vi "SVFA Zoom Power Spectral Density (N Ch).vi"(0 "scaled signals [EU]":waveform(dbl)[](array[waveform]), 3 "zoom settings":T2={"frequency range"={"start frequency"=1000.0, "stop frequency"=2000.0}, "window"=1, "number of lines"=400, "% overlap"=0.0} {"% overlap" min=0.0 format="%.2f"; "number of lines" min=2; "window" items=["None ", "Hanning", "Hamming", "Blackman-Harris", "Exact Blackman", "Blackman", "Flat Top", "4 Term B-Harris ", "7 Term B-Harris", "Low Sidelobe"]; "frequency range"."stop frequency" min=0.0 format="%.2f"; "frequency range"."start frequency" min=0.0 format="%.2f"}, 4 "dB On (T)":bool=TRUE, 5 "error in (no error)":errorcluster, 6 "desired units":enum16{"EU^2 / Hz", "EU / sqrt(Hz)"}(ring), 7 "averaging parameters":T1={"averaging mode"=enum."No averaging", "weighting mode"=enum."Exponential", "number of averages"=10, "linear mode"=enum."One shot"} {"number of averages" min=1 step=1}, 9 "restart averaging (F)":bool) -> (11 "averaging done":bool, 12 "new spectrum available":bool, 13 "averages completed":dbl, 14 "power spectral densities [EU^2 rms / Hz]":cluster{"f0":dbl, "df":dbl, "magnitude":dbl[]}[](array[cluster]) {"magnitude" format="%.2p"; "df" format="%.2p"; "f0" format="%.2p"}, 15 "unit labels":string[](array[string]), 18 "spectrum info":T3[](array[typedef]) {"x-axis units" items=["Time (s)"=0, "Frequency-CB (Hz)"=1, "Frequency-CPB (Hz)"=1248, "Frequency-Arbitrary (Hz)"=2357, "Quefrency (s)"=2, "Revolutions (rev)"=3, "Order"=4, "Speed (RPM)"=11, "Speed (rad/s)"=21, "Index"=65535]; "weighting filter" items=["Linear", "A-weighting", "B-weighting", "C-weighting", "ITU-R 468-4", "Dolby", "CCITT", "C-message", "Wb", "Wc", "Wd", "We", "Wf", "Wh", "Wj", "Wk", "Wm", "AES17 20 kHz lowpass", "AES17 40 kHz lowpass", "AES17 20 kHz highpass", "AES17 40 kHz highpass"]; "dB reference [EU]" format="%.2f"; "engineering units" items=["custom..."=0, "V"=1, "A"=21, "C"=30, "pC"=31, "s"=32, "-"=29, "Pa"=2, "N"=20, "g"=3, "m/s^2"=4, "m/s"=5, "m"=6, "mm/s"=12, "mm"=13, "micron/s"=14, "micron"=15, "in/s^2"=7, "in/s"=8, "in"=9, "mil/s"=10, "mil"=11, "rad/s^2"=16, "rad/s"=17, "rad"=18, "deg/s^2"=26, "deg/s"=27, "deg"=28, "RPM"=22, "cycle/s^2"=23, "Hz"=24, "cycle"=25, "strain"=19]; "spectral info"."window" items=["None "=0, "Hanning"=1, "Hamming"=2, "Blackman-Harris"=3, "Exact Blackman"=4, "Blackman"=5, "Flat Top"=6, "4 Term B-Harris "=7, "7 Term B-Harris"=8, "Low Sidelobe"=9, "Force - Exponential"=10, "Gaussian"=62]}, 19 "error out":errorcluster)   [LabVIEW 2017]
doc: "Computes the zoom power spectral density of <B>scaled signal [EU]</B> and <B>zoom settings</B>. Data accumulates each time this VI is called. However, it returns a new spectrum only when sufficient data accumulates. Indicators and subsequent processing should only be called when <B>new spectrum available</B> is TRUE. Wire data to the <B>scaled signal [EU]</B> input to determine the polymorphic instance to use or manually select the instance."
uses:
  <vilib>/addons/_NISVFA/_Shared subVIs/Controls/svc_Spectrum Info.ctl
  <vilib>/addons/_NISVFA/_Shared subVIs/Controls/svc_X-Axis Units.ctl
  <vilib>/addons/_NISVFA/_Shared subVIs/Controls/svc_Spectrum Type.ctl
  <vilib>/addons/_NISVFA/_Shared subVIs/Controls/svc_Engineering Units Text Ring.ctl
  <vilib>/addons/_NISVFA/_Shared subVIs/Controls/svc_Weighting Filter Text Ring.ctl
  <vilib>/addons/_NISVFA/_Shared subVIs/Controls/svc_Complimentary Spectrum Units.ctl
  <vilib>/addons/_NISVFA/_Shared subVIs/Spectrum Info/svfa_Build Spectrum Info.vi
  <vilib>/addons/_NISVFA/_Shared subVIs/Spectrum Averaging/svfa_Reset Averaging State Info.vi
  <vilib>/addons/_NISVFA/_Shared subVIs/Spectrum Averaging/svfa_Average Array with Avg Checks (complex) No State.vi
  <vilib>/addons/_NISVFA/_Shared subVIs/Common/svc_Complex to Mag2 Array.vi
  <vilib>/addons/_NISVFA/_Shared subVIs/Spectrum Averaging/svfa_Average Array with Avg Checks (real) No State.vi
  <vilib>/addons/_NISVFA/_Shared subVIs/Common/svc_Get SV Channel Info.vi
  <vilib>/addons/_NISVFA/_Shared subVIs/Common/svc_Spectrum Units.vi
  <vilib>/addons/_NISVFA/_Shared subVIs/Spectrum Averaging/svfa_Average Array (complex) No State.vi
  <vilib>/addons/_NISVFA/_Shared subVIs/Spectrum Averaging/svfa_Average Array (real) No State.vi
  <vilib>/addons/_NISVFA/_Shared subVIs/Spectrum Averaging/svfa_No Average Array (complex).vi
  <vilib>/addons/_NISVFA/_Shared subVIs/Spectrum Averaging/svfa_Average Array (complex).vi
  <vilib>/addons/_NISVFA/_Shared subVIs/Spectrum Averaging/svfa_No Average Array (real).vi
  <vilib>/addons/_NISVFA/_Shared subVIs/Spectrum Averaging/svfa_Average Array (real).vi
  <vilib>/addons/_NISVFA/_Shared subVIs/Spectrum Averaging/svfa_Peak Hold Array.vi
  <vilib>/addons/_NISVFA/_Spectrum Processing/SVFA Unit Conversion (N Ch).vi
  <vilib>/addons/_NISVFA/_Shared subVIs/Common/svc_Get Weighting Enum and Labels.vi
  <vilib>/addons/_NISVFA/_Shared subVIs/Common/svc_Unit Label Lexical Class.vi
  <vilib>/addons/_NISVFA/_Shared subVIs/Common/svc_Engineering Units to Unit Label.vi
  <vilib>/addons/_NISVFA/_Shared subVIs/Common/svc_Format Value (DBL).vi
  <vilib>/addons/_NISVFA/_Shared subVIs/Common/svc_Channel Info to Spectrum Info.vi
  <vilib>/addons/_NISVFA/_Shared subVIs/Common/svc_Unit Label to Engineering Units.vi
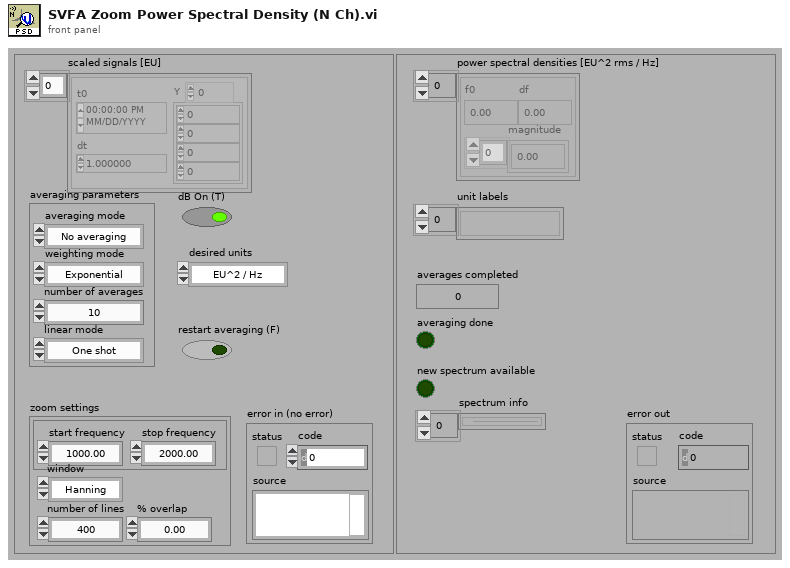
[diagram p1: front panel]
types:
  T1 = cluster{"averaging mode":enum16{"No averaging", "Vector averaging", "RMS averaging", "Peak hold"}, "weighting mode":enum16{"Linear", "Exponential"}, "number of averages":u32, "linear mode":enum16{"One shot", "Auto restart"}}
  T2 = cluster{"frequency range":cluster{"start frequency":dbl, "stop frequency":dbl}, "window":u16, "number of lines":i32, "% overlap":dbl}
  T3 = typedef "svc_Spectrum Info.ctl" = cluster{"channel name":string, "description":string, "x-axis units":T4, "spectral info":cluster{"spectrum type":T5, "linear/dB":enum16{"linear", "dB"}, "window":u16, "window size":i32, "FFT size":i32}, "engineering units":T6, "custom label":string, "dB reference [EU]":dbl, "peak units":enum16{"rms", "peak", "peak-peak"}, "weighting filter":T7, "spectral density?":bool, "unit label":string, "spectrum skewed?":bool, "complimentary spectrum units":T8}
  T4 = typedef "svc_X-Axis Units.ctl" = u16
  T5 = typedef "svc_Spectrum Type.ctl" = enum16{"FFT Spectrum [complex]", "Amplitude [Magnitude]", "Power [Magnitude^2]", "Cross Spectrum [complex]", "Frequency Response [Complex]"}
  T6 = typedef "svc_Engineering Units Text Ring.ctl" = u16
  T7 = typedef "svc_Weighting Filter Text Ring.ctl" = u16
  T8 = typedef "svc_Complimentary Spectrum Units.ctl" = enum16{"none", "radians", "degrees", "cycles", "imaginary"}
  T9 = enum16{"Restart processing", "Continue processing", "Skip processing"}
  T10 = enum16{"No averaging", "Vector averaging", "RMS averaging", "Peak hold"}
  T11 = cluster{"linear/dB":enum16{"no change", "linear", "dB"}, "dB reference (0: no change)":dbl, "power/magnitude":enum16{"no change", "power", "magnitude"}, "view":enum16{"no change", "rms", "peak", "peak-peak"}}
  T12 = enum16{"no change", "spectrum", "spectral density"}
  T13 = cluster{"zoom settings":cluster{"center frequency":dbl, "zoom":i32, "trim":dbl}, "FFT settings":cluster{"window":enum16{"None ", "Hanning", "Hamming", "Blackman-Harris", "Exact Blackman", "Blackman", "Flat Top", "4 Term B-Harris ", "7 Term B-Harris", "Low Sidelobe"}, "window size":i32, "FFT size":i32, "%overlap":dbl}}
  T14 = cluster{"complex FFT":cdb[], "real FFT":dbl[], "f0":dbl, "df":dbl, "averages completed":dbl, "averaging parameters":cluster{"averaging mode":enum16{"No averaging", "Vector averaging", "RMS averaging", "Peak hold"}, "weighting mode":enum16{"Linear", "Exponential"}, "number of averages":u32, "linear mode":enum16{"One shot", "Auto restart"}}}[]
  T15 = cluster{"complex FFT":cdb[], "real FFT":dbl[], "f0":dbl, "df":dbl, "averages completed":dbl, "averaging parameters":cluster{"averaging mode":enum16{"No averaging", "Vector averaging", "RMS averaging", "Peak hold"}, "weighting mode":enum16{"Linear", "Exponential"}, "number of averages":u32, "linear mode":enum16{"One shot", "Auto restart"}}}
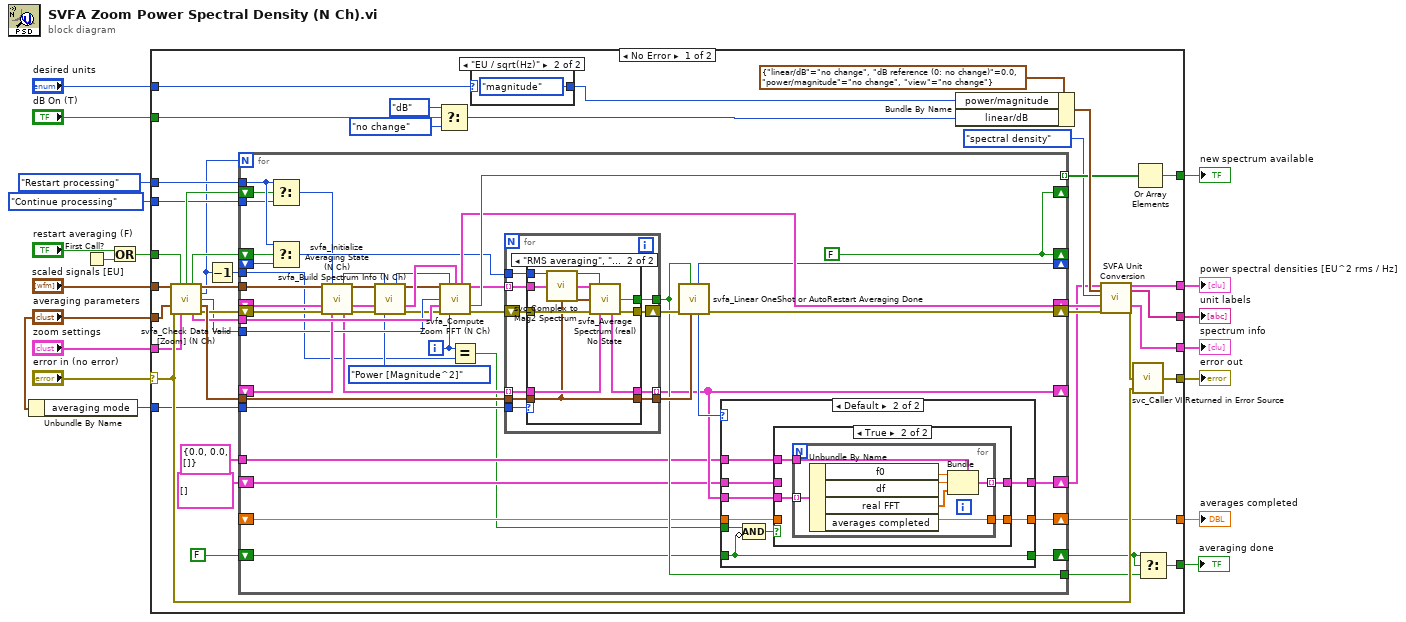
[diagram p0: block diagram]
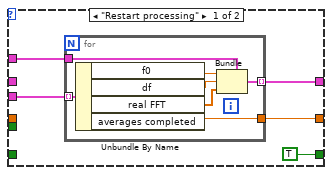
[diagram p2: hidden frame]
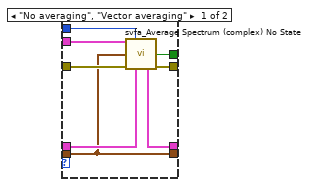
[diagram p4: hidden frame]
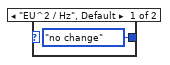
[diagram p5: hidden frame]
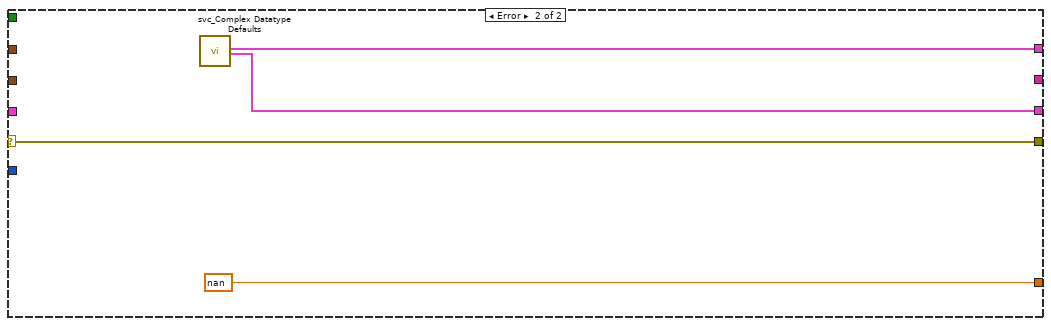
[diagram p6: hidden frame]
diagram:
  n1 = Unbundle By Name("averaging parameters") -> ("averaging mode"=w1:T10)
  n2 = First Call?() -> (First Call?: T/F=w8:bool)
  n3 = Or(x="restart averaging (F)", y=w8) -> (x .or. y?=w6:bool)
  n4 = case shown="No Error" "error in (no error)" {
    selector: "error in (no error)" -> [w52 w175]
    tunnel: w6 -> [w34 _]
    tunnel: [w24 nan ("Averaged So-far")] -> w19
    tunnel: [w35 _] -> w18
    tunnel: [w62 w172] -> w14
    tunnel: [w58 w175] -> w17
    tunnel: "averaging parameters" -> [w39 _]
    tunnel: "zoom settings" -> [w38 _]
    tunnel: "scaled signals [EU]" -> [w51 _]
    tunnel: [w60 _] -> w13
    tunnel: "dB On (T)" -> [w44 _]
    tunnel: [w59 w173] -> w12
    tunnel: [w23 _] -> w10
    tunnel: "desired units" -> [w45 _]
    tunnel: T9."Restart processing" ("processing control in") -> [w33 _]
    tunnel: T9."Continue processing" ("processing control in") -> [w31 _]
    tunnel: w1 -> [w28 _]
    frame No Error {
      n5 = call <vilib>:"svfa_Check Data Valid [Zoom] (N Ch).vi"("scaled signals [EU]"=w51, "restart averaging (F)"=w34, "averaging parameters"=w39, "error in (no error)"=w52, "zoom settings"=w38) -> ("reset processing"=w32:bool, "restart averaging"=w53:bool, "dup scaled signals"=w57:waveform(dbl)[], "iterations"=w30:i32, "maximum block size"=w36:i32, "dup averaging parameters"=w56:T1, "zoom FFT settings"=w54:T13, "error out"=w55:errorcluster)  [unwired: 3 in]
      n6 = Decrement(x=w30) -> (x-1=w29:i32)
      n7 = for {
        N: w30 -> [_]
        tunnel: [w105] -> w42 mode=indexing
        tunnel: w54 -> [w107]
        tunnel: w57 -> [w108]
        tunnel: [w74] -> w22
        shift-left: _ -> [w101]
        shift-right: [w72] -> _
        shift-right: [w103] -> w41
        shift-left: _ -> [w102]
        tunnel: w56 -> [w100]
        shift-right: [w73] -> _
        shift-left: _ -> [w99]
        tunnel: w33 -> [w95]
        tunnel: w36 -> [w96]
        shift-right: [w63] -> _
        shift-left: w53 -> [w97]
        tunnel: w31 -> [w93]
        tunnel: w29 -> [w78]
        tunnel: w28 -> [w76]
        shift-right: [w104] -> w40
        shift-left: w55 -> [w106]
        shift-right: [w63] -> _
        shift-left: w32 -> [w94]
        tunnel: cluster{"f0":dbl, "df":dbl, "real FFT":dbl[]} {"f0"=0.0, "df"=0.0, "real FFT"=[]} ("cluster") -> [w71]
        shift-right: [w65] -> w21
        shift-left: cluster{"f0":dbl, "df":dbl, "real FFT":dbl[]}[] [] -> [w70]
        shift-right: [w66] -> w20
        shift-left: FALSE ("restart averaging") -> [w67]
        shift-right: [w69] -> w24
        shift-left: _ -> [w68]
        i -> [w77]
        w63 = FALSE ("restart averaging")
        n8 = Select(t=w95, s=w94, f=w93) -> (s? t:f=w79:T9)
        n9 = Select(t=w95, s=w97, f=w99) -> (s? t:f=w98:T9)
        n10 = call <vilib>:"svfa_Initialize Averaging State (N Ch).vi"("Windowed Waveform(s)"=w108, "processing control in"=w79, "spectra info in"=w102, "error in (no error)"=w106, "state info"=w101) -> ("processing control out"=w87:T9, "Windowed Waveform(s)"=w86:waveform(dbl)[], "spectra info out"=w84:T3[], "state info"=w83:T14, "error out"=w85:errorcluster)  [unwired: 6 in]
        n11 = call <vilib>:"svfa_Build Spectrum Info (N Ch).vi"("scaled signal(s)"=w86, "processing control in"=w87, "spectra info in"=w84, "error in (no error)"=w85, "spectrum type"=svc_Spectrum_Type."Power [Magnitude^2]") -> ("dup processing control"=w80:T9, "dup scaled signals"=w89:waveform(dbl)[], "spectra info out"=w91:T3[], "error out"=w81:errorcluster)  [unwired: 7 in]
        n12 = call <vilib>:"svfa_Compute Zoom FFT (N Ch).vi"("scaled signals [EU]"=w89, "processing control"=w80, "spectra info in"=w91, "maximum block size"=w96, "zoom FFT settings"=w107, "error in (no error)"=w81, "iteration"=w77) -> ("spectra info out"=w103:T3[], "FFT spectra"=w88:cluster{"f0":dbl, "df":dbl, "spectrum":cdb[]}[], "spectrum ready"=w105:bool, "error out"=w90:errorcluster)  [unwired: 4 in, 1 out]
        n13 = Equal?(x=w77, y=w78) -> (x = y?=w64:bool)
        n14 = for {
          tunnel: [w152] -> w74
          tunnel: w88 -> [w151] mode=indexing
          tunnel: w98 -> [w148]
          tunnel: w100 -> [w147]
          tunnel: w76 -> [w146]
          tunnel: w83 -> [w145] mode=indexing
          tunnel: [w144] -> w72 mode=indexing
          shift-right: [w149] -> w92
          shift-left: w90 -> [w150]
          tunnel: [w143] -> w75
          n15 = case shown="\"RMS averaging\", \"Peak hold\"" w146 {
            tunnel: w147 -> [w153 w161]
            tunnel: [w158 w167] -> w149
            tunnel: [w157 w168] -> w152
            tunnel: w151 -> [w160 w166]
            tunnel: w150 -> [w159 w169]
            tunnel: w148 -> [w156 w164]
            tunnel: w145 -> [w155 w162]
            tunnel: [w154 w163] -> w144
            tunnel: [w153 w161] -> w143
            frame "No averaging", "Vector averaging" {
              n16 = call <vilib>:"svfa_Average Spectrum (complex) No State.vi"("spectrum"=w160, "processing control"=w156, "averaging parameters"=w153, "error in (no error)"=w159, "averaging state info in"=w155) -> ("averaging done"=w157:bool, "averaging state info out"=w154:T15, "error out"=w158:errorcluster)  [unwired: 5 in, 3 out]
            }
            frame "RMS averaging", "Peak hold" {
              n17 = call <vilib>:"svc_Complex to Mag2 Spectrum.vi"("complex spectrum"=w166) -> ("power spectrum"=w165:cluster{"f0":dbl, "df":dbl, "spectrum":dbl[]})  [unwired: 4 in]
              n18 = call <vilib>:"svfa_Average Spectrum (real) No State.vi"("spectrum"=w165, "processing control"=w164, "averaging parameters"=w161, "error in (no error)"=w169, "averaging state info in"=w162) -> ("averaging done"=w168:bool, "averaging state info out"=w163:T15, "error out"=w167:errorcluster)  [unwired: 5 in, 3 out]
            }
          }
        }
        n19 = call <vilib>:"svfa_Linear OneShot or AutoRestart Averaging Done.vi"("averaging parameters"=w75, "averaging done"=w74, "error in (no error)"=w92) -> ("error out"=w104:errorcluster, "processing control"=w73:T9)  [unwired: 7 in]
        n20 = case shown="Default" w73 {
          tunnel: w72 -> [w113 w129]
          tunnel: [TRUE ("restart averaging") w124] -> w66
          tunnel: [w111 w128] -> w65
          tunnel: w67 -> [_ w124]
          tunnel: w64 -> [_ w127]
          tunnel: w71 -> [w110 w126]
          tunnel: [w109 w123] -> w69
          tunnel: w68 -> [_ w122]
          tunnel: w70 -> [_ w121]
          frame "Restart processing" {
            n21 = for {
              tunnel: w113 -> [w117] mode=indexing
              tunnel: [w116] -> w111 mode=indexing
              tunnel: w110 -> [w115]
              tunnel: [w114] -> w109
              n22 = Unbundle By Name(w117) -> ("f0"=w120:dbl, "df"=w119:dbl, "real FFT"=w118:dbl[], "averages completed"=w114:dbl)
              n23 = Bundle(cluster=w115, "f0"=w120, "df"=w119, "real FFT"=w118) -> (w116:cluster{"f0":dbl, "df":dbl, "real FFT":dbl[]})
            }
          }
          frame Default {
            n24 = Compound Arithmetic op=AND(w127, invert w124) -> (w125:bool)
            n25 = case shown="True" w125 {
              tunnel: w129 -> [_ w135]
              tunnel: [w130 w134] -> w128
              tunnel: w126 -> [_ w133]
              tunnel: [w131 w132] -> w123
              tunnel: w122 -> [w131 _]
              tunnel: w121 -> [w130 _]
              frame False {
              }
              frame True {
                n26 = for {
                  tunnel: w135 -> [w139] mode=indexing
                  tunnel: [w138] -> w134 mode=indexing
                  tunnel: w133 -> [w137]
                  tunnel: [w136] -> w132
                  n27 = Unbundle By Name(w139) -> ("f0"=w142:dbl, "df"=w141:dbl, "real FFT"=w140:dbl[], "averages completed"=w136:dbl)
                  n28 = Bundle(cluster=w137, "f0"=w142, "df"=w141, "real FFT"=w140) -> (w138:cluster{"f0":dbl, "df":dbl, "real FFT":dbl[]})
                }
              }
            }
          }
        }
      }
      n29 = Select(t=enum16{"no change", "linear", "dB"}."dB" ("linear/dB"), s=w44, f=enum16{"no change", "linear", "dB"}."no change" ("linear/dB")) -> (s? t:f=w48:enum16{"no change", "linear", "dB"})
      n30 = case shown="\"EU / sqrt(Hz)\"" w45 {
        tunnel: [enum16{"no change", "power", "magnitude"}."no change" ("power/magnitude") enum16{"no change", "power", "magnitude"}."magnitude" ("power/magnitude")] -> w50
        frame "EU^2 / Hz", Default {
        }
        frame "EU / sqrt(Hz)" {
        }
      }
      n31 = Bundle By Name(cluster=T11 {"linear/dB"=enum."no change", "dB reference (0: no change)"=0.0, "power/magnitude"=enum."no change", "view"=enum."no change"} ("desired scaling"), "power/magnitude"=w50, "linear/dB"=w48) -> (w43:T11)
      n32 = call-poly <vilib>:"SVFA Unit Conversion.vi"("spectra"=w21, "desired scaling"=w43, "spectral density desired"=T12."spectral density", "spectrum info in"=w41, "error in (no error)"=w40) -> ("converted spectra"=w62:cluster{"x0":dbl, "dx":dbl, "magnitude":dbl[]}[], "unit labels"=w60:string[], "spectrum info out"=w59:T3[], "error out"=w61:errorcluster)  [unwired: 11 in]
      n33 = call <vilib>:"svc_Caller VI Returned in Error Source.vi"("warning input to caller"=w52, "error in (no error)"=w61) -> ("error out"=w58:errorcluster)  [unwired: 3 in]
      n34 = Or Array Elements(Boolean array=w42) -> (logical OR=w35:bool)
      n35 = Select(t=w20, s=w20, f=w22) -> (s? t:f=w23:bool)
    }
    frame Error {
      n36 = call <vilib>:"svc_Complex Datatype Defaults.vi"() -> ("empty array of spectra"=w172:cluster{"f0":dbl, "df":dbl, "magnitude":dbl[]}[], "empty array of spectrum info"=w173:T3[])  [unwired: 11 in, 7 out]
    }
  }
  "averages completed" <- w19
  "new spectrum available" <- w18
  "error out" <- w17
  "power spectral densities [EU^2 rms / Hz]" <- w14
  "unit labels" <- w13
  "spectrum info" <- w12
  "averaging done" <- w10
